vi "Extract Image Data Y.vi"(4 "Negative Slope":bool, 6 "Averaged Values":dbl[][](array[numeric]), 7 "Detector Interval":i32=5, 8 "Original values":dbl[](array[numeric]), 9 "Grouped Arrays":dbl[](array[numeric]), 10 "Bounding Box":cluster{dbl, dbl, dbl, dbl, dbl}, 11 "String":string) -> (2 "Centerpoint":cluster{dbl, dbl})   [LabVIEW 2018]
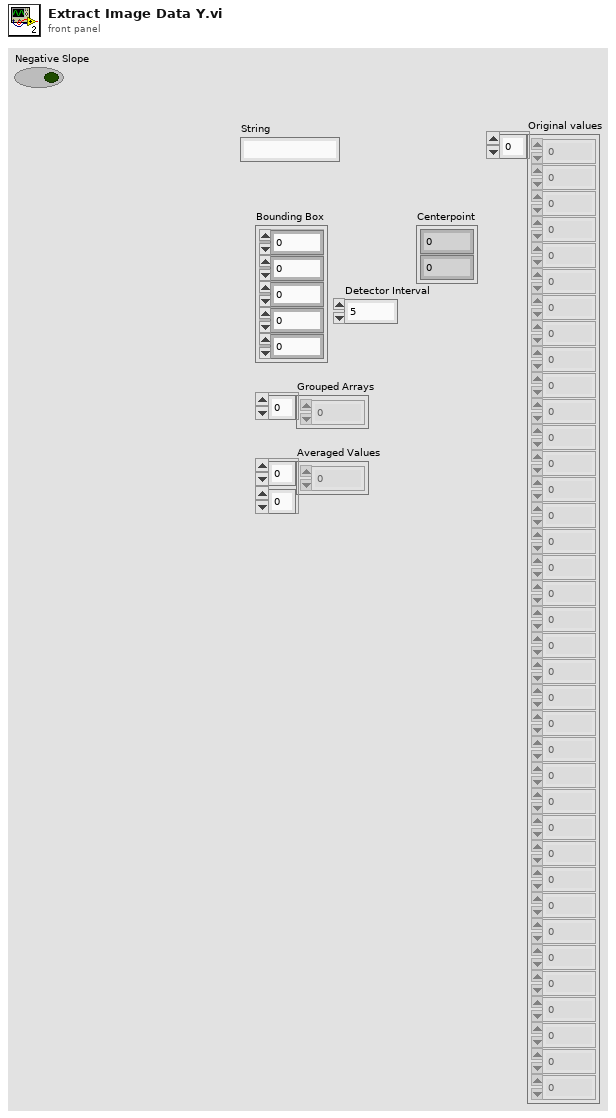
[diagram p1: front panel]
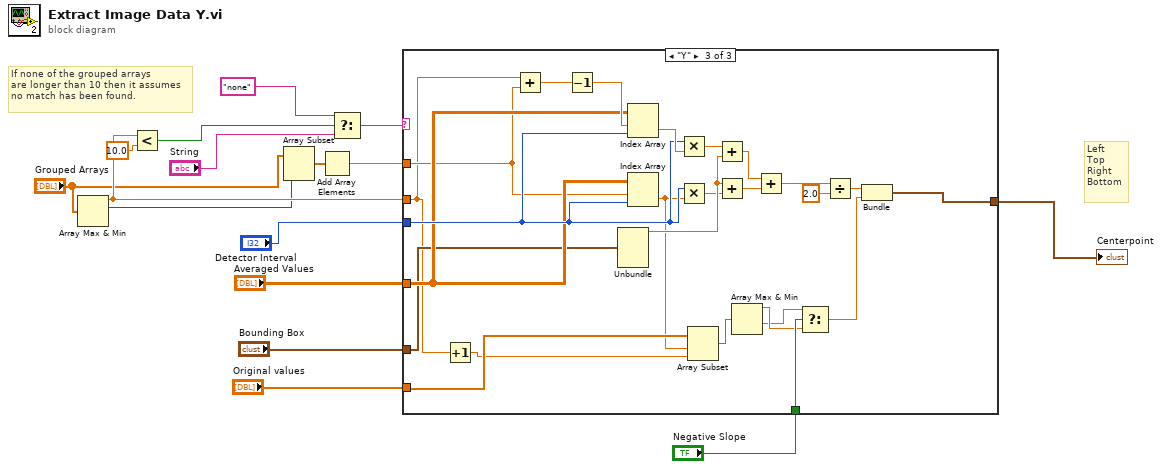
[diagram p0: block diagram]
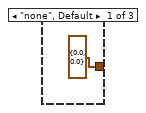
[diagram p2: hidden frame]
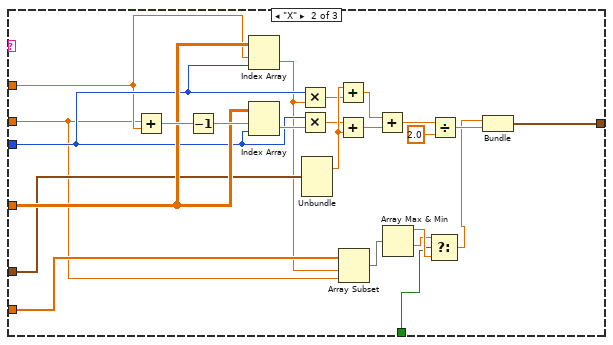
[diagram p3: hidden frame]
diagram:
  # "If none of the grouped arrays\nare longer than 10 then it assumes\nno match has been found."
  # "Left\nTop\nRight\nBottom"
  n1 = Array Max & Min(array="Grouped Arrays") -> (max value=w15:dbl, max index (indices)=w3:i32)  [unwired: 2 out]
  n2 = Less?(x=w15, y=10.0) -> (x < y?=w13:bool)
  n3 = Array Subset(array="Grouped Arrays", length=w3) -> (w5:dbl[])  [unwired: 1 in]
  n4 = Add Array Elements(numeric array=w5) -> (sum=w2:dbl)
  n5 = Select(t="none", s=w13, f="String") -> (s? t:f=w10:string)
  n6 = case shown="\"Y\"" w10 {
    tunnel: w15 -> [_ w22 w48]
    tunnel: [cluster{dbl, dbl} {0.0, 0.0} w30 w55] -> w16
    tunnel: "Original values" -> [_ w28 w54]
    tunnel: "Detector Interval" -> [_ w26 w52]
    tunnel: "Averaged Values" -> [_ w27 w51]
    tunnel: "Bounding Box" -> [_ w25 w50]
    tunnel: w2 -> [_ w24 w49]
    tunnel: "Negative Slope" -> [_ w18 w45]
    frame "none", Default {
    }
    frame "X" {
      n7 = Add(x=w22, y=w24) -> (x+y=w36:dbl)
      n8 = Decrement(x=w36) -> (x-1=w35:dbl)
      n9 = Index Array(array=w27, index (row)=w24, index (col)=w26) -> (element=w23:dbl)
      n10 = Index Array(array=w27, index (row)=w35, index (col)=w26) -> (element=w32:dbl)
      n11 = Multiply(x=w26, y=w23) -> (x*y=w34:dbl)
      n12 = Multiply(x=w26, y=w32) -> (x*y=w33:dbl)
      n13 = Unbundle(w25) -> (w37:dbl)  [unwired: 4 out]
      n14 = Add(x=w37, y=w34) -> (x+y=w39:dbl)
      n15 = Add(x=w33, y=w37) -> (x+y=w40:dbl)
      n16 = Array Subset(array=w28, index=w23, length=w22) -> (w29:dbl[])
      n17 = Add(x=w39, y=w40) -> (x+y=w38:dbl)
      n18 = Array Max & Min(array=w29) -> (max value=w20:dbl, min value=w19:dbl)  [unwired: 2 out]
      n19 = Select(t=w19, s=w18, f=w20) -> (s? t:f=w21:dbl)
      n20 = Divide(x=w38, y=2.0) -> (x/y=w41:dbl)
      n21 = Bundle(w21, w41) -> (w30:cluster{dbl, dbl})  [unwired: 1 in]
    }
    frame "Y" {
      n22 = Increment(x=w48) -> (x+1=w47:dbl)
      n23 = Add(x=w48, y=w49) -> (x+y=w58:dbl)
      n24 = Decrement(x=w58) -> (x-1=w59:dbl)
      n25 = Unbundle(w50) -> (w65:dbl)  [unwired: 4 out]
      n26 = Index Array(array=w51, index (row)=w59, index (col)=w52) -> (element=w62:dbl)
      n27 = Index Array(array=w51, index (row)=w49, index (col)=w52) -> (element=w46:dbl)
      n28 = Multiply(x=w52, y=w62) -> (x*y=w61:dbl)
      n29 = Multiply(x=w52, y=w46) -> (x*y=w60:dbl)
      n30 = Array Subset(array=w54, index=w46, length=w47) -> (w53:dbl[])
      n31 = Add(x=w61, y=w65) -> (x+y=w57:dbl)
      n32 = Add(x=w65, y=w60) -> (x+y=w56:dbl)
      n33 = Array Max & Min(array=w53) -> (max value=w44:dbl, min value=w43:dbl)  [unwired: 2 out]
      n34 = Add(x=w57, y=w56) -> (x+y=w63:dbl)
      n35 = Select(t=w43, s=w45, f=w44) -> (s? t:f=w42:dbl)
      n36 = Divide(x=w63, y=2.0) -> (x/y=w66:dbl)
      n37 = Bundle(w66, w42) -> (w55:cluster{dbl, dbl})  [unwired: 1 in]
    }
  }
  "Centerpoint" <- w16
